vi "ReadComicCache.vi"(8 "error in (no error)":errorcluster, 11 "Comics in":refnum<class "Comics.lvclass">) -> (0 "error out":errorcluster, 3 "Comics out":refnum<class "Comics.lvclass">)   [LabVIEW 2022 SP3, in "Comics.lvclass"]
uses:
  Comics.lvclass
  TypeDefs/Comic.ctl
  TypeDefs/Character.ctl
  TypeDefs/Creator.ctl
  TypeDefs/Variant.ctl
  Comics.lvclass/Comics.ctl
  <vilib>/Utility/cursorutil.llb/Set Cursor (Icon Pict).vi
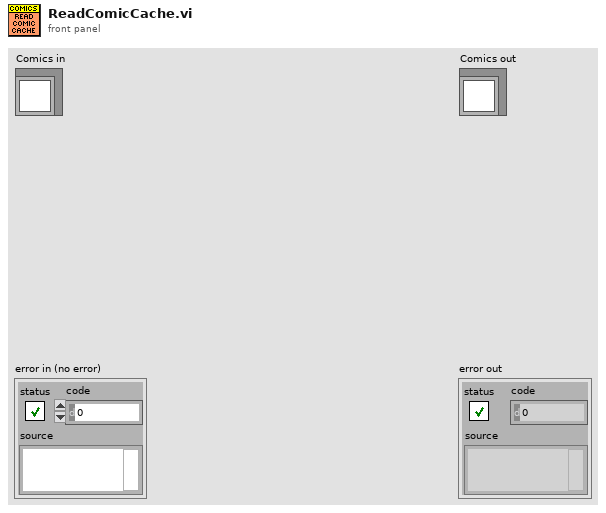
[diagram p1: front panel]
types:
  T1 = typedef "Comic.ctl" = cluster{"URL":string, "Series URL":string, "Series":string, "Volume":i32, "Issue":string, "Title":string, "Description":string, "Page Count":i32, "Cover Price":dbl, "UPC":string, "Characters":T2[], "Creators":T3[], "Main Cover URL":string, "Variant Covers":T4[], "DatePublished":timestamp}
  T2 = typedef "Character.ctl" = cluster{"Name":string, "Real-Name":string, "Universe":string, "URL":string}
  T3 = typedef "Creator.ctl" = cluster{"Name":string, "URL":string, "Creator Types":string[]}
  T4 = typedef "Variant.ctl" = cluster{"URL":string, "Description":string, "Cover URL":string}
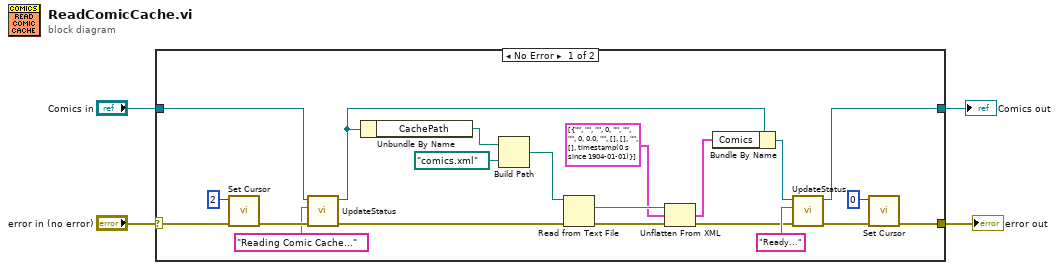
[diagram p0: block diagram]
diagram:
  n1 = case shown="No Error" "error in (no error)" {
    selector: "error in (no error)" -> [w22 w27]
    tunnel: [w21 w27] -> w3
    tunnel: [w15 w26] -> w1
    tunnel: "Comics in" -> [w20 w26]
    frame No Error {
      n2 = call-poly <vilib>:"Set Cursor.vi"("error in (no error)"=w22, "icon"=u16 2) -> ("error out"=w19:errorcluster)  [unwired: 8 in, 1 out]
      n3 = call "UpdateStatus.vi"("error in (no error)"=w19, "Status"="Reading Comic Cache...", "Comics in"=w20) -> ("error out"=w18:errorcluster, "Comics out"=w9:refnum<class "Comics.lvclass">)  [unwired: 7 in]
      n4 = Unbundle By Name(w9) -> ("CachePath"=w25:path)
      n5 = Build Path(base path=w25, name or relative path=path "comics.xml") -> (appended path=w23:path)
      n6 = Read from Text File(file (use dialog)=w23, error in=w18) -> (text=w11:string, error out=w13:errorcluster)  [unwired: 2 in, 2 out]
      n7 = Unflatten From XML(xml string=w11, type=T1[] [{"URL"="", "Series URL"="", "Series"="", "Volume"=0, "Issue"="", "Title"="", "Description"="", "Page Count"=0, "Cover Price"=0.0, "UPC"="", "Characters"=[], "Creators"=[], "Main Cover URL"="", "Variant Covers"=[], "DatePublished"=timestamp(0 s since 1904-01-01)}], error in (no error)=w13) -> (value=w8:T1[], error out=w12:errorcluster)
      n8 = Bundle By Name(cluster=w9, "Comics"=w8) -> (w7:refnum<class "Comics.lvclass">)
      n9 = call "UpdateStatus.vi"("error in (no error)"=w12, "Status"="Ready...", "Comics in"=w7) -> ("error out"=w14:errorcluster, "Comics out"=w15:refnum<class "Comics.lvclass">)  [unwired: 7 in]
      n10 = call-poly <vilib>:"Set Cursor.vi"("error in (no error)"=w14, "icon"=u16 0) -> ("error out"=w21:errorcluster)  [unwired: 8 in, 1 out]
    }
    frame Error {
    }
  }
  "error out" <- w3
  "Comics out" <- w1
